vi "CB Test HoloDrive.vi"() -> ()   [LabVIEW 2020]
uses:
  State-Space/CB State Space.ctl
  <vilib>/Analysis/Matrix/Datatypes/RealMatrix.ctl
  <vilib>/Analysis/Matrix/NI_Matrix.lvlib
panel:
  out "K (gain matrix)":T1
  in  "r":dbl[](array[numeric])=[40.0, 40.0, 720.0] format="%.2f"
  in  "q":dbl[](array[numeric])=[0.5, 0.5, 4.0] format="%.2f"
  out "Discrete SSM":T2
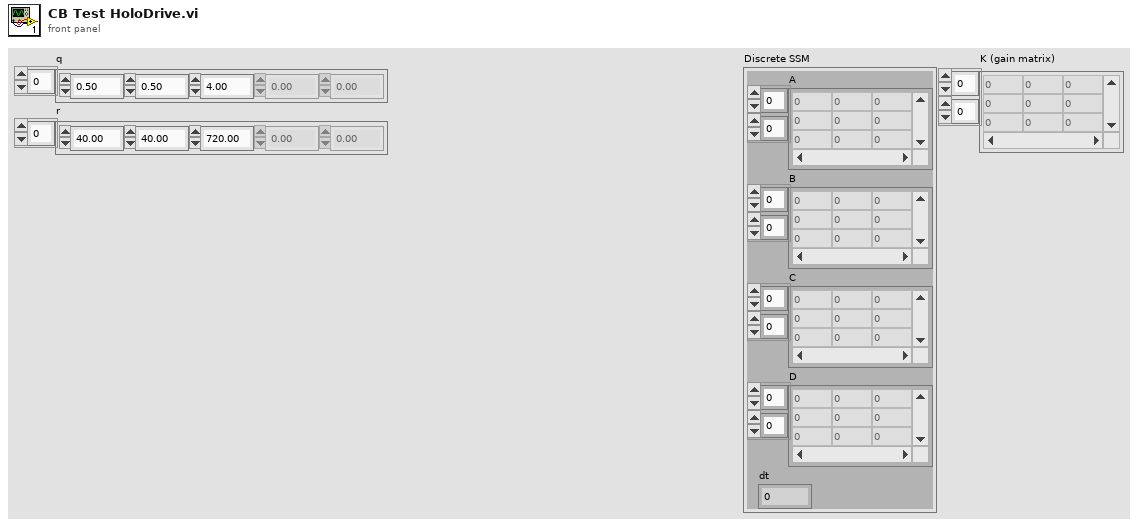
[diagram p1: front panel]
types:
  T1 = typedef "NI_Matrix.lvlib/RealMatrix.ctl" = dbl[][]
  T2 = typedef "CB State Space.ctl" = cluster{"A":T1, "B":T1, "C":T1, "D":T1, "dt":dbl}
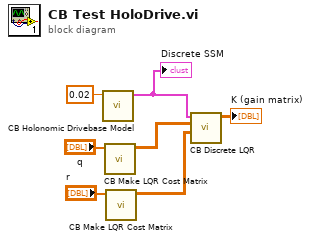
[diagram p0: block diagram]
diagram:
  n1 = call "CB Holonomic Drivebase Model.vi"("dt"=0.02) -> ("Discrete SSM"=w6:T2)  [unwired: 10 in]
  "Discrete SSM" <- w6
  n2 = call "CB Make LQR Cost Matrix.vi"("q"="q") -> ("Q"=w3:T1)  [unwired: 10 in]
  n3 = call "CB Make LQR Cost Matrix.vi"("q"="r") -> ("Q"=w2:T1)  [unwired: 10 in]
  n4 = call "CB Discrete LQR.vi"("R"=w2, "Q"=w3, "State Space Model"=w6) -> ("K (gain matrix)"=→"K (gain matrix)":T1)  [unwired: 7 in, 1 out]
